vi "ex_GetChNames.vi"(1 "Signals":waveform(dbl)[](array[waveform])) -> (0 "Channel Names":string[](array[string]))   [LabVIEW 2020]
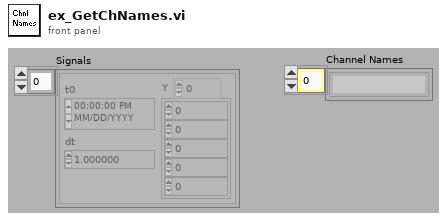
[diagram p1: front panel]
types:
  T1 = typedef "ex_WaveformAttribs.ctl" = cluster{"Start Timestamp":timestamp, "Timestamp":timestamp, "Relative Time?":bool, "X Dimension":string, "Signal Name":string}
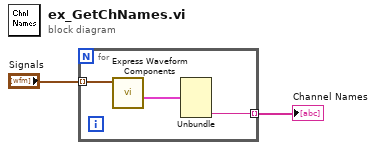
[diagram p0: block diagram]
diagram:
  n1 = for {
    tunnel: "Signals" -> [w4] mode=indexing
    tunnel: [w3] -> w1 mode=indexing
    n2 = call <vilib>:"Express Waveform Components.vi"("Waveform"=w4) -> ("Express Waveform Attributes"=w5:T1)  [unwired: 1 in, 9 out]
    n3 = Unbundle(w5) -> ("Signal Name"=w3:string)  [unwired: 4 out]
  }
  "Channel Names" <- w1
